vi "Fdx Create Tx Queue Data Frame.vi"(6 "UDPsrcPort":u16, 7 "UDPdstPort":u16, 8 "error in":errorcluster, 9 "Payload":u8[](array[numeric])=[1, 2, 3, 4, 0, 0, 0, 0, 0, 0, 0, 0, 0, 0, 0, 0, 0, 0, 0, 0, 0, 0, 0, 0, 0, 0, 0, 0, 0, 0, 0, 0, 0, 0, 0, 0, 0, 0, 0, 0, 0, 0, 0, 0, 1, 0, 0, 0, 0, 0, 0, 0, 0, 0, 0, 0, 0, 0, 0, 0, 0, 0, 0, 0, 0, 0, 0, 0, 0, 0, 0, 0, 0, 0, 0, 0, 0, 0, 0, 0, 0, 0, 0, 0, 0, 0, 0, 0, 0, 0, 0, 0, 0, 0, 0, 0, 0, 0, 0, 1] format="%.0x", 10 "afdx configuration":T1={"domainID"=1, "sideID"=1, "locationID"=1, "interfaceID"=1, "partitionID"=1} {"interfaceID" format="%.0b"}, 11 "VL Id":u16=60) -> (0 "error out":errorcluster, 3 "Frame":u8[](array[numeric])=[1, 2, 3, 4, 0, 0, 0, 0, 0, 0, 0, 0, 0, 0, 0, 0, 0, 0, 0, 0, 0, 0, 0, 0, 0, 0, 0, 0, 0, 0, 0, 0, 0, 0, 0, 0, 0, 0, 0, 0, 0, 0, 0, 0, 1, 0, 0, 0, 0, 0, 0, 0, 0, 0, 0, 0, 0, 0, 0, 0, 0, 0, 0, 0, 0, 0, 0, 0, 0, 0, 0, 0, 0, 0, 0, 0, 0, 0, 0, 0, 0, 0, 0, 0, 0, 0, 0, 0, 0, 0, 0, 0, 0, 0, 0, 0, 0, 0, 0, 1] format="%.0x")   [LabVIEW 2020, in "AIM664LV.lvlib"]
uses:
  AIM664LV.lvlib
  _controls/queue_data_full.ctl
  helpers/EthFrameManagement/controls/IPFrame_type.ctl
  helpers/EthFrameManagement/controls/UDPFrame_type.ctl
  helpers/EthFrameManagement/controls/mac_src_info_afdx.ctl
  helpers/EthFrameManagement/controls/ehternetFrame_type.ctl
  helpers/EthFrameManagement/controls/ip_src_info_afdx.ctl
  helpers/EthFrameManagement/EthFrameManagement.lvlib
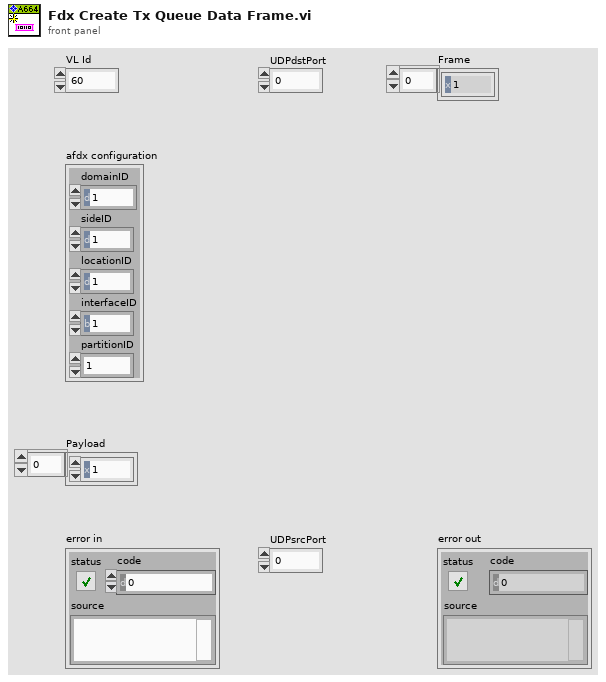
[diagram p1: front panel]
types:
  T1 = typedef "AIM664LV.lvlib/queue_data_full.ctl" = cluster{"domainID":u8, "sideID":u8, "locationID":u8, "interfaceID":u8, "partitionID":u8}
  T2 = typedef "EthFrameManagement.lvlib/ip_src_info_afdx.ctl" = cluster{"domainID":u8, "sideID":u8, "locationID":u8, "partitionID":u8}
  T3 = typedef "EthFrameManagement.lvlib/ehternetFrame_type.ctl" = cluster{"Dest MAC":u8[], "Src MAC":u8[], "EtherType":u16}
  T4 = typedef "EthFrameManagement.lvlib/mac_src_info_afdx.ctl" = cluster{"domainID":u8, "sideID":u8, "locationID":u8, "interfaceID":u8}
  T5 = typedef "EthFrameManagement.lvlib/UDPFrame_type.ctl" = cluster{"Source Port":u16, "Dest Port":u16, "Lenght":u16, "Checksum":u16}
  T6 = typedef "EthFrameManagement.lvlib/IPFrame_type.ctl" = cluster{"Version":u8, "IHL":u8, "QoS":u8, "Lenght":u16, "ID":u16, "FragOffset":u16, "TTL":u8, "Protocol":u8, "Checksum":u16, "Source IP":u32, "Dest IP":u32}
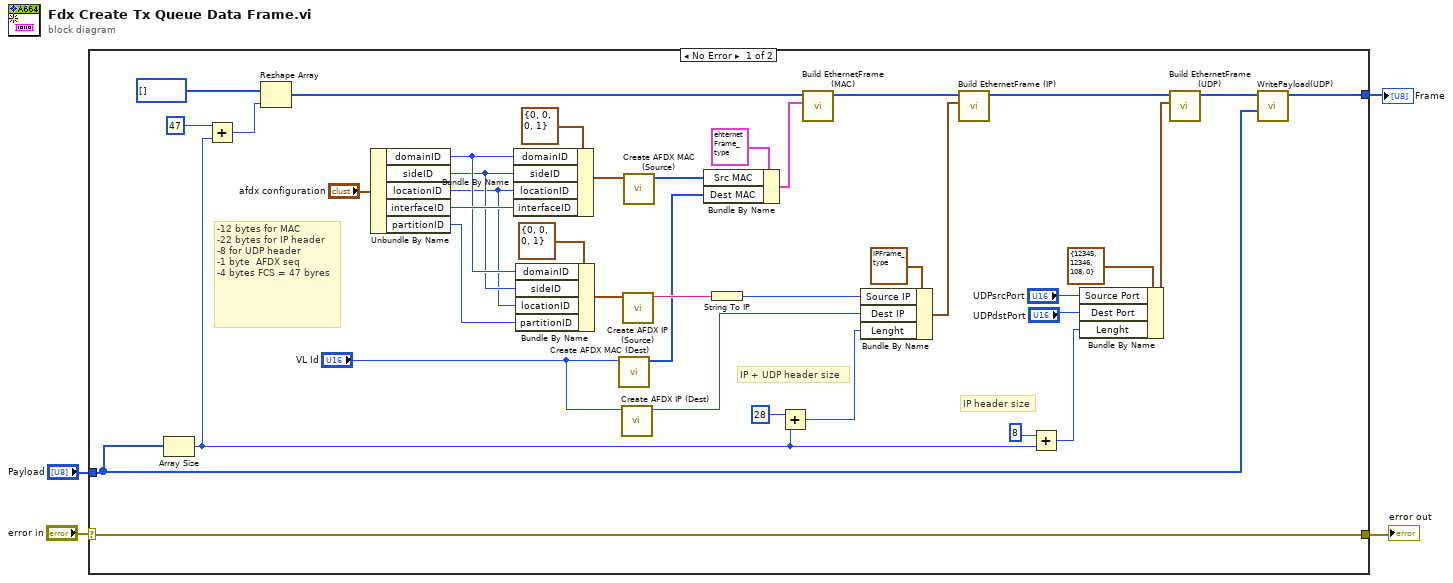
[diagram p0: block diagram]
diagram:
  n1 = case shown="No Error" "error in" {
    selector: "error in" -> [w5 w44]
    tunnel: "Payload" -> [w42 _]
    tunnel: [w29 _] -> w3
    tunnel: [w5 w44] -> w1
    frame No Error {
      # "-12 bytes for MAC\n-22 bytes for IP header\n-8 for UDP header\n-1 byte  AFDX seq\n-4 bytes FCS = 47 byres"
      # "IP header size"
      # "IP + UDP header size"
      n2 = Array Size(array=w42) -> (size(s)=w12:i32)
      n3 = Add(x=47, y=w12) -> (x+y=w11:i32)
      n4 = Reshape Array(u8[] [] ("Payload 2"), w11) -> (w9:u8[])
      n5 = Unbundle By Name("afdx configuration") -> ("domainID"=w34:u8, "sideID"=w33:u8, "locationID"=w32:u8, "interfaceID"=w37:u8, "partitionID"=w31:u8)
      n6 = Bundle By Name(cluster=T4 {"domainID"=0, "sideID"=0, "locationID"=0, "interfaceID"=1} ("Source Info"), "domainID"=w34, "sideID"=w33, "locationID"=w32, "interfaceID"=w37) -> (w39:T4)
      n7 = Bundle By Name(cluster=T2 {"domainID"=0, "sideID"=0, "locationID"=0, "partitionID"=1} ("Source Info"), "domainID"=w34, "sideID"=w33, "locationID"=w32, "partitionID"=w31) -> (w35:T2)
      n8 = call "Create AFDX MAC (Dest).vi"("VL Id"="VL Id") -> ("MAC-src"=w8:u8[])  [unwired: 10 in]
      n9 = call "Create AFDX IP (Dest).vi"("VL"="VL Id") -> ("ip net"=w6:u32)  [unwired: 9 in, 1 out]
      n10 = call "Create AFDX IP (Source).vi"("Source Info"=w35) -> ("ip address"=w30:string)  [unwired: 10 in]
      n11 = call "Create AFDX MAC (Source).vi"("Source Info"=w39) -> ("MAC-src"=w18:u8[])  [unwired: 10 in]
      n12 = Bundle By Name(cluster=T3 {"Dest MAC"=[3, 0, 0, 0, 0, 60], "Src MAC"=[2, 0, 0, 1, 33, 32], "EtherType"=2048} ("MAC header"), "Src MAC"=w18, "Dest MAC"=w8) -> (w40:T3)
      n13 = String To IP(1:w30) -> (0:w19:u32)
      n14 = Add(x=28, y=w12) -> (x+y=w16:i32)
      n15 = call "Build EthernetFrame (MAC).vi"("MAC header"=w40, "Ethernet Frame In"=w9) -> ("Ethernet Frame Out"=w25:u8[])  [unwired: 9 in]
      n16 = Bundle By Name(cluster=T6 {"Version"=4, "IHL"=5, "QoS"=0, "Lenght"=128, "ID"=0, "FragOffset"=16384, "TTL"=1, "Protocol"=17, "Checksum"=0, "Source IP"=0, "Dest IP"=0} ("IP header"), "Source IP"=w19, "Dest IP"=w6, "Lenght"=w16) -> (w20:T6)
      n17 = call "Build EthernetFrame (IP).vi"("IP header"=w20, "Ethernet Frame In"=w25) -> ("Ethernet Frame Out"=w27:u8[])  [unwired: 9 in]
      n18 = Add(x=8, y=w12) -> (x+y=w14:i32)
      n19 = Bundle By Name(cluster=T5 {"Source Port"=12345, "Dest Port"=12346, "Lenght"=108, "Checksum"=0} ("UDP header"), "Source Port"="UDPsrcPort", "Dest Port"="UDPdstPort", "Lenght"=w14) -> (w23:T5)
      n20 = call "Build EthernetFrame (UDP).vi"("UDP header"=w23, "Ethernet Frame In"=w27) -> ("Ethernet Frame Out"=w24:u8[])  [unwired: 9 in]
      n21 = call "WritePayload(UDP).vi"("Payload"=w42, "Ethernet Frame In"=w24) -> ("Ethernet Frame Out"=w29:u8[])  [unwired: 9 in]
    }
    frame Error {
    }
  }
  "Frame" <- w3
  "error out" <- w1
